vi "Process Output.vi"(0 "RMXPowerSupply in":refnum<class "RMXPowerSupply.lvclass">, 9 "AdasLvTemplate in":refnum<class "AdasLvTemplate.lvclass">, 11 "error in":errorcluster) -> (3 "ErrorCode":i32, 4 "RMXPowerSupply out":refnum<class "RMXPowerSupply.lvclass">, 6 "Output Status":i32, 8 "Current":dbl, 10 "AdasLvTemplate out":refnum<class "AdasLvTemplate.lvclass">, 13 "Running Status":i32, 14 "Voltage to Write":dbl, 15 "error out":errorcluster)   [LabVIEW 2023]
uses:
  <vilib>/ADAS Replay HIL/ADAS Plugin Utilities/AdasLvTemplate/AdasLvTemplate.lvclass
  <vilib>/ADAS Replay HIL/ADAS Plugin Utilities/AdasLvTemplate/Typedefs/Out Of Band/Status Custom U64 Selector.ctl
  <vilib>/ADAS Replay HIL/ADAS Plugin Utilities/AdasLvTemplate/Typedefs/Out Of Band/Status Custom DBL Selector.ctl
  Support/Class/RMXPowerSupply.lvclass
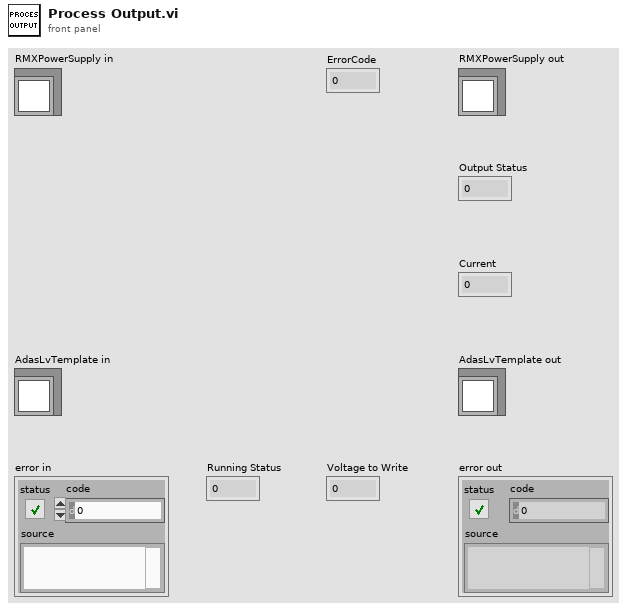
[diagram p1: front panel]
types:
  T1 = typedef "AdasLvTemplate.lvlib/AdasLvTemplate.lvclass/Status Custom DBL Selector.ctl" = enum16{"Custom 5 (DBL)", "Custom 6 (DBL)", "Custom 7 (DBL)", "Custom 8 (DBL)"}
  T2 = typedef "AdasLvTemplate.lvlib/AdasLvTemplate.lvclass/Status Custom U64 Selector.ctl" = enum16{"Custom 1 (U64)", "Custom 2 (U64)", "Custom 3 (U64)", "Custom 4 (U64)"}
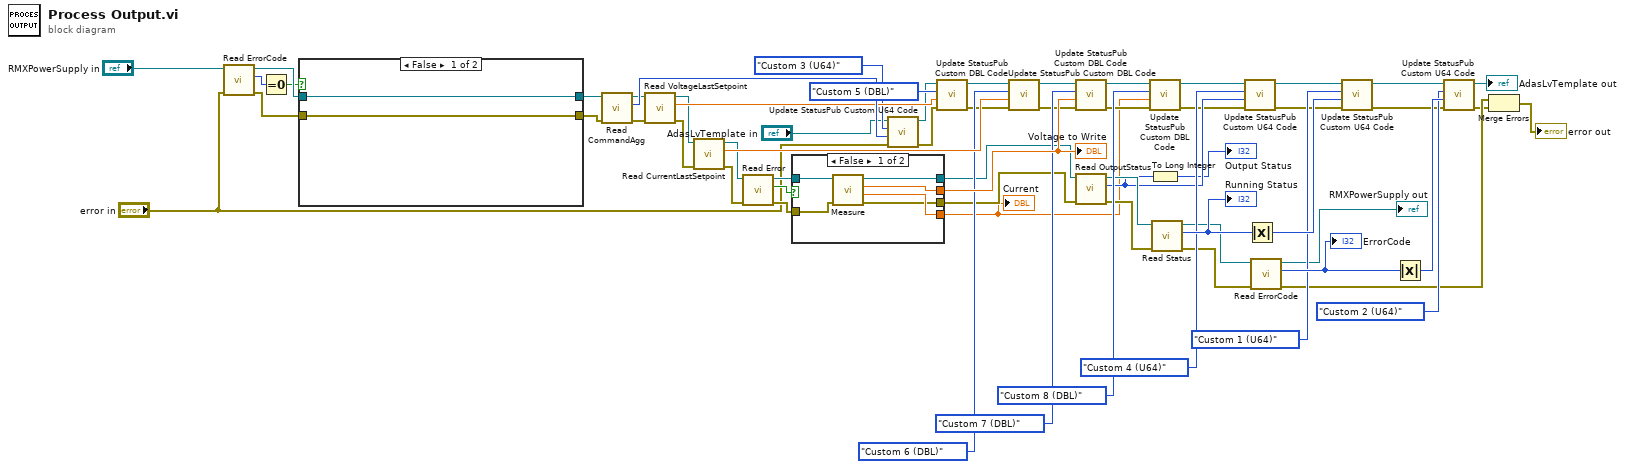
[diagram p0: block diagram]
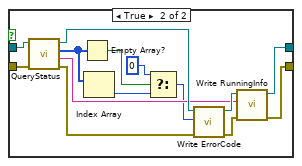
[diagram p2: hidden frame]
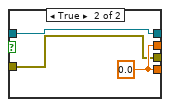
[diagram p3: hidden frame]
diagram:
  n1 = call-dynamic "Read ErrorCode.vi"("error in (no error)"="error in", "RMXPowerSupply in"="RMXPowerSupply in") -> ("error out"=w20:errorcluster, "ErrorCode"=w18:i32, "RMXPowerSupply out"=w21:refnum<class "RMXPowerSupply.lvclass">)  [unwired: 7 in]
  n2 = Equal To 0?(x=w18) -> (x = 0?=w19:bool)
  n3 = case shown="False" w19 {
    tunnel: w21 -> [w64 w78]
    tunnel: w20 -> [w63 w77]
    tunnel: [w63 w72] -> w24
    tunnel: [w64 w71] -> w23
    frame False {
    }
    frame True {
      n4 = call-dynamic "QueryStatus.vi"("error in (no error)"=w77, "RMXPowerSupply in"=w78) -> ("error out"=w75:errorcluster, "Error Message"=w70:string, "Error Code"=w69:i32[], "RMXPowerSupply out"=w76:refnum<class "RMXPowerSupply.lvclass">)  [unwired: 6 in]
      n5 = Empty Array?(array=w69) -> (empty?=w68:bool)
      n6 = Index Array(array=w69) -> (element=w65:i32)  [unwired: 1 in]
      n7 = Select(t=0, s=w68, f=w65) -> (s? t:f=w66:i32)
      n8 = call-dynamic "Write ErrorCode.vi"("error in (no error)"=w75, "ErrorCode"=w66, "RMXPowerSupply in"=w76) -> ("error out"=w73:errorcluster, "RMXPowerSupply out"=w74:refnum<class "RMXPowerSupply.lvclass">)  [unwired: 7 in]
      n9 = call-dynamic "Write RunningInfo.vi"("error in (no error)"=w73, "RunningInfo"=w70, "RMXPowerSupply in"=w74) -> ("error out"=w72:errorcluster, "RMXPowerSupply out"=w71:refnum<class "RMXPowerSupply.lvclass">)  [unwired: 7 in]
    }
  }
  n10 = call-dynamic "Read CommandAgg.vi"("error in (no error)"=w24, "RMXPowerSupply in"=w23) -> ("error out"=w61:errorcluster, "CommandAgg"=w62:u64, "RMXPowerSupply out"=w60:refnum<class "RMXPowerSupply.lvclass">)  [unwired: 7 in]
  n11 = call-dynamic "Read VoltageLastSetpoint.vi"("error in (no error)"=w61, "RMXPowerSupply in"=w60) -> ("error out"=w52:errorcluster, "VoltageLastSetpoint"=w54:dbl, "RMXPowerSupply out"=w51:refnum<class "RMXPowerSupply.lvclass">)  [unwired: 7 in]
  n12 = call-dynamic "Read CurrentLastSetpoint.vi"("error in (no error)"=w52, "RMXPowerSupply in"=w51) -> ("error out"=w28:errorcluster, "CurrentLastSetpoint"=w53:dbl, "RMXPowerSupply out"=w29:refnum<class "RMXPowerSupply.lvclass">)  [unwired: 7 in]
  n13 = call-dynamic "Read Error.vi"("error in (no error)"=w28, "RMXPowerSupply in"=w29) -> ("error out"=w26:errorcluster, "Error"=w25:bool, "RMXPowerSupply out"=w27:refnum<class "RMXPowerSupply.lvclass">)  [unwired: 7 in]
  n14 = case shown="False" w25 {
    tunnel: [w84 w87] -> w3
    tunnel: [w83 w87] -> w50
    tunnel: [w82 w85] -> w33
    tunnel: [w81 w86] -> w31
    tunnel: w27 -> [w80 w86]
    tunnel: w26 -> [w79 w85]
    frame False {
      n15 = call-dynamic "Measure.vi"("error in (no error)"=w79, "RMXPowerSupply in"=w80) -> ("error out"=w82:errorcluster, "Current"=w84:dbl, "Voltage"=w83:dbl, "RMXPowerSupply out"=w81:refnum<class "RMXPowerSupply.lvclass">)  [unwired: 5 in, 1 out]
    }
    frame True {
      w87 = 0.0 ("Voltage")
    }
  }
  "Voltage to Write" <- w50
  "Current" <- w3
  n16 = call <vilib>:"Update StatusPub Custom U64 Code.vi"("error in (no error)"="error in", "Custom Data"=w62, "Terminal"=Status_Custom_U64_Selector."Custom 3 (U64)", "AdasLvTemplate in"="AdasLvTemplate in") -> ("error out"=w12:errorcluster, "AdasLvTemplate out"=w11:refnum<class "AdasLvTemplate.lvclass">)  [unwired: 6 in]
  n17 = call <vilib>:"Update StatusPub Custom DBL Code.vi"("error in (no error)"=w12, "Custom Data"=w54, "Terminal"=Status_Custom_DBL_Selector."Custom 5 (DBL)", "AdasLvTemplate in"=w11) -> ("error out"=w43:errorcluster, "AdasLvTemplate out"=w44:refnum<class "AdasLvTemplate.lvclass">)  [unwired: 6 in]
  n18 = call <vilib>:"Update StatusPub Custom DBL Code.vi"("error in (no error)"=w43, "Custom Data"=w53, "Terminal"=Status_Custom_DBL_Selector."Custom 6 (DBL)", "AdasLvTemplate in"=w44) -> ("error out"=w8:errorcluster, "AdasLvTemplate out"=w9:refnum<class "AdasLvTemplate.lvclass">)  [unwired: 6 in]
  n19 = call <vilib>:"Update StatusPub Custom DBL Code.vi"("error in (no error)"=w8, "Custom Data"=w50, "Terminal"=Status_Custom_DBL_Selector."Custom 7 (DBL)", "AdasLvTemplate in"=w9) -> ("error out"=w42:errorcluster, "AdasLvTemplate out"=w45:refnum<class "AdasLvTemplate.lvclass">)  [unwired: 6 in]
  n20 = call-dynamic "Read OutputStatus.vi"("error in (no error)"=w33, "RMXPowerSupply in"=w31) -> ("error out"=w32:errorcluster, "OutputStatus"=w22:u8, "RMXPowerSupply out"=w30:refnum<class "RMXPowerSupply.lvclass">)  [unwired: 7 in]
  n21 = call <vilib>:"Update StatusPub Custom DBL Code.vi"("error in (no error)"=w42, "Custom Data"=w3, "Terminal"=Status_Custom_DBL_Selector."Custom 8 (DBL)", "AdasLvTemplate in"=w45) -> ("error out"=w6:errorcluster, "AdasLvTemplate out"=w7:refnum<class "AdasLvTemplate.lvclass">)  [unwired: 6 in]
  n22 = To Long Integer(number=w22) -> (32bit integer=→"Output Status":i32)
  n23 = call-dynamic "Read Status.vi"("error in (no error)"=w32, "RMXPowerSupply in"=w30) -> ("error out"=w35:errorcluster, "Status"=w56:i32, "RMXPowerSupply out"=w34:refnum<class "RMXPowerSupply.lvclass">)  [unwired: 7 in]
  "Running Status" <- w56
  n24 = call <vilib>:"Update StatusPub Custom U64 Code.vi"("error in (no error)"=w6, "Custom Data"=w22, "Terminal"=Status_Custom_U64_Selector."Custom 4 (U64)", "AdasLvTemplate in"=w7) -> ("error out"=w4:errorcluster, "AdasLvTemplate out"=w5:refnum<class "AdasLvTemplate.lvclass">)  [unwired: 6 in]
  n25 = Absolute Value(x=w56) -> (abs(x)=w57:i32)
  n26 = call-dynamic "Read ErrorCode.vi"("error in (no error)"=w35, "RMXPowerSupply in"=w34) -> ("error out"=w36:errorcluster, "ErrorCode"=w58:i32, "RMXPowerSupply out"=→"RMXPowerSupply out":refnum<class "RMXPowerSupply.lvclass">)  [unwired: 7 in]
  "ErrorCode" <- w58
  n27 = call <vilib>:"Update StatusPub Custom U64 Code.vi"("error in (no error)"=w4, "Custom Data"=w57, "Terminal"=Status_Custom_U64_Selector."Custom 1 (U64)", "AdasLvTemplate in"=w5) -> ("error out"=w15:errorcluster, "AdasLvTemplate out"=w14:refnum<class "AdasLvTemplate.lvclass">)  [unwired: 6 in]
  n28 = Absolute Value(x=w58) -> (abs(x)=w59:i32)
  n29 = call <vilib>:"Update StatusPub Custom U64 Code.vi"("error in (no error)"=w15, "Custom Data"=w59, "Terminal"=Status_Custom_U64_Selector."Custom 2 (U64)", "AdasLvTemplate in"=w14) -> ("error out"=w17:errorcluster, "AdasLvTemplate out"=→"AdasLvTemplate out":refnum<class "AdasLvTemplate.lvclass">)  [unwired: 6 in]
  n30 = Merge Errors(w36, w17) -> (→"error out":errorcluster)
